vi "Global_ACT_Data Out.vi"() -> ()   [LabVIEW 2020, in "Arm_ACT.lvlib"]
uses:
  Arm_ACT.lvlib
panel:
  out "Wrist Level":bool
  out "At Target":bool
  in  "ACT_Template_CycleTime(S)":dbl
  # "The Names of the Data items in the Global Variable MUST describe who the Single Writer is\nFor Actuator Globals the the naming convention is\n   \nACT_Lib Name_Data Name\n\nExamples:\nACT_Drive_X axis\nACT_Hopper_AgitatorSpeed"
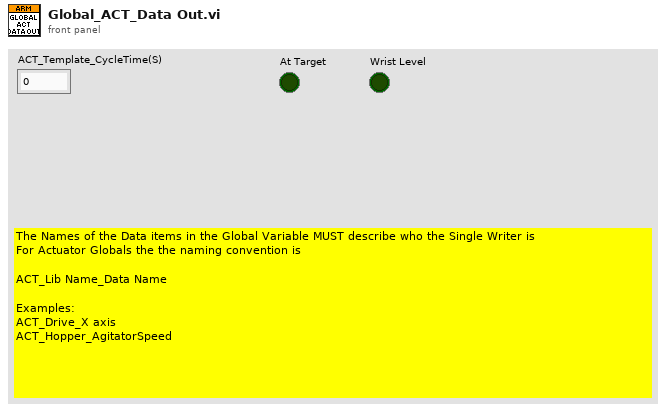
[diagram p1: front panel]
diagram:
